vi "Treat Command.vi"(8 "error in (no error)":errorcluster, 11 "Channel in":refnum<class "ECHARPE_Channel.lvclass">) -> (0 "error out":errorcluster, 3 "Channel out":refnum<class "ECHARPE_Channel.lvclass">)   [LabVIEW 2018, in "ECHARPE_Channel.lvclass"]
doc: "Treat the commando received from the control interface."
uses:
  ECHARPE_Channel.lvclass
  C:/Users/Denis/Desktop/S4ACS/S4ACS/Channel/Channel.lvclass
  Channel/Channel.lvclass/Channel.ctl
  RxTx/RxTx.lvclass
  State Machine/State Machine.lvclass
  Sim_CCD/Sim_CCD.lvclass
  Channel/Channel.lvclass
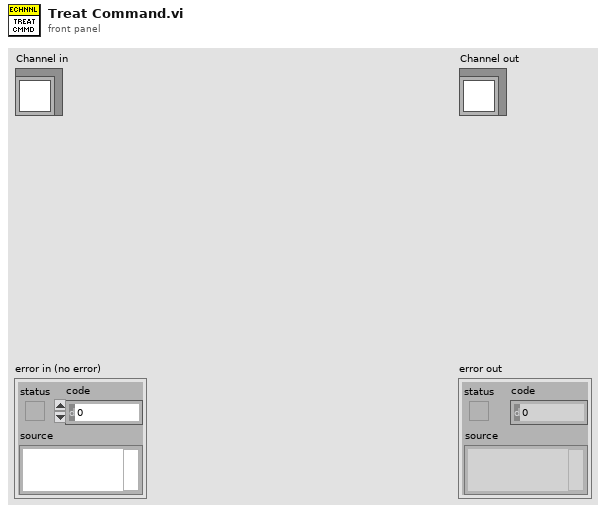
[diagram p1: front panel]
types:
  T1 = cluster{"State Machine.lvclass":refnum<class "State Machine.lvclass">, "RxTx.lvclass":refnum<class "RxTx.lvclass">, "Save_Header_RxTx.lvclass":refnum<class "RxTx.lvclass">, "Status SM.lvclass":refnum<class "State Machine.lvclass">, "Status RxTx.lvclass":refnum<class "RxTx.lvclass">, "servers array":refnum<class "Server.lvclass">[], "Events log file.lvclass":refnum<class "Log File.lvclass">, "Errors log file.lvclass":refnum<class "Log File.lvclass">, "Keywords log file.lvclass":refnum<class "Log File.lvclass">, "Sim_CCD.lvclass":refnum<class "Sim_CCD.lvclass">}
  T2 = cluster{"field 1":string, "field 2":string, "field 3":string}
  T3 = cluster{"Stop Acquisition":bool, "Abort Acquisition":bool, "Pause acquisition":bool, "wait expose command":bool, "video mode":bool, "stop app":bool}
  T4 = cluster{"FRAMES_DONE":u16, "CCD_STATUS":string, "CURRENT_TEMPERATURE":i16, "TEMPERATURE_STATUS":string, "FRAME_EXPOSURE_TIME":dbl, "SERIAL_NUMBER":u16, "ACQUIRING":bool, "POWER":bool, "ACS MODE":bool}
  T5 = cluster{"CYCLES_DONE":u16, "LAST_IMAGE_NAME":string, "USED_DISK_SPACE":u16, "IMAGE_INDEX":u32, "acquisition error":bool}
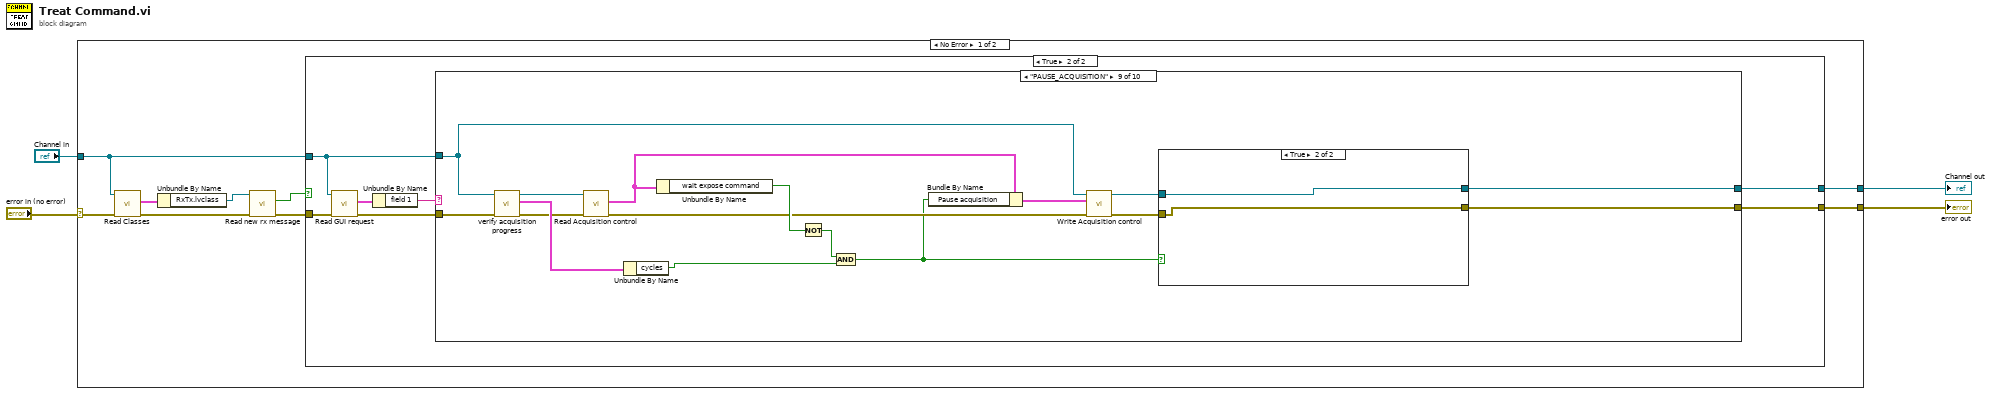
[diagram p0: block diagram]
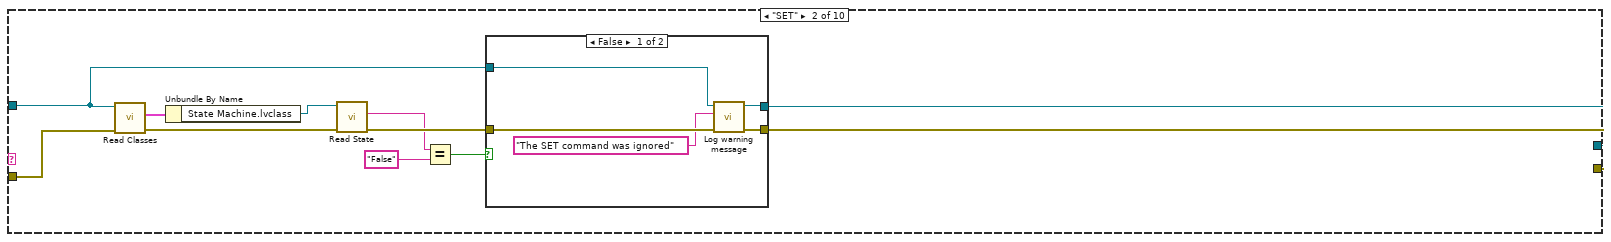
[diagram p4: hidden frame]
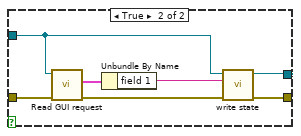
[diagram p5: hidden frame]
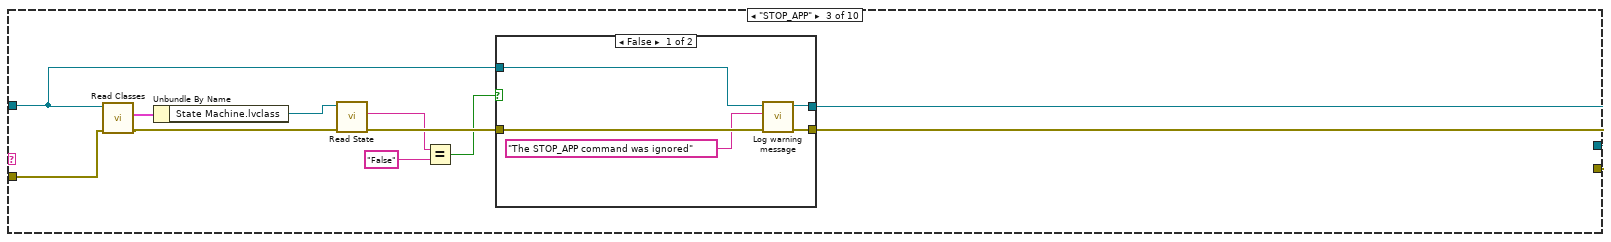
[diagram p6: hidden frame]
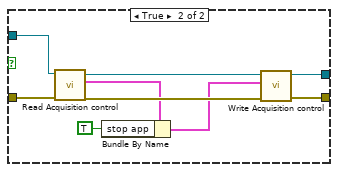
[diagram p7: hidden frame]
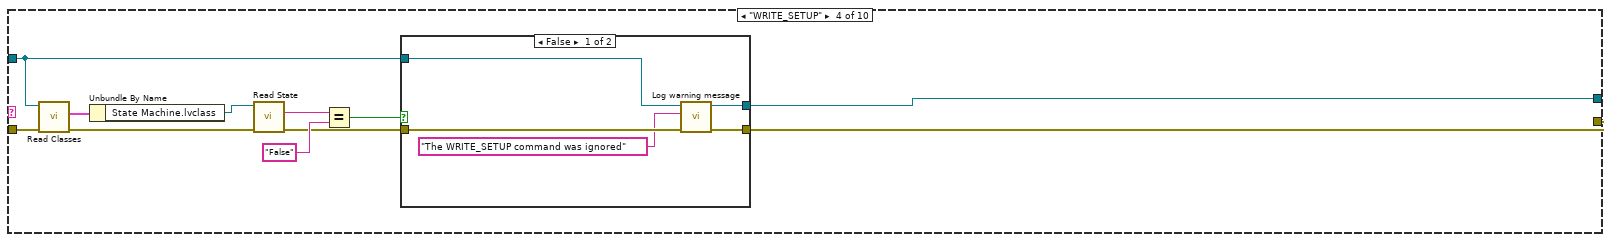
[diagram p8: hidden frame]
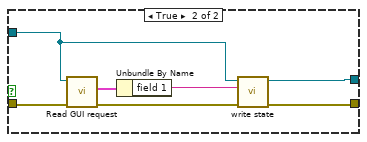
[diagram p9: hidden frame]
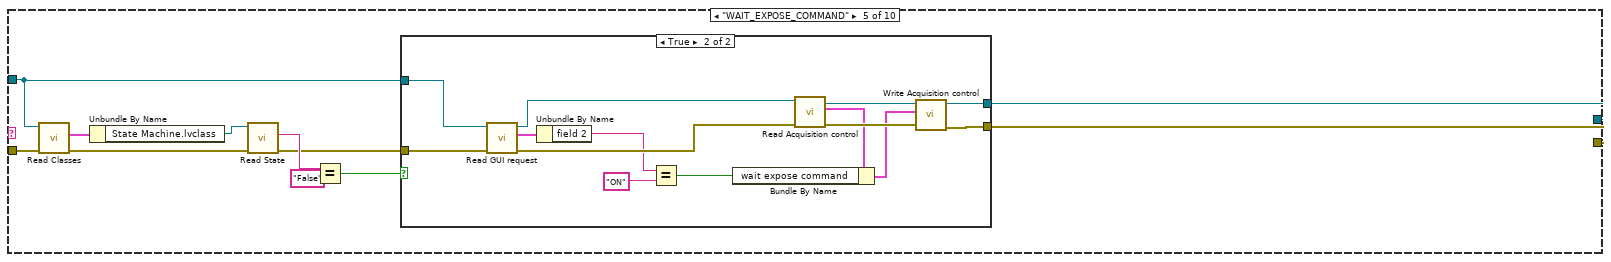
[diagram p10: hidden frame]
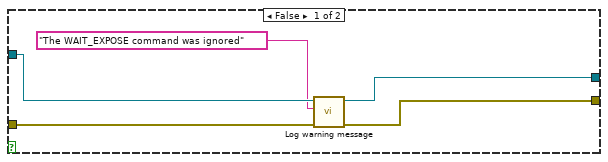
[diagram p11: hidden frame]
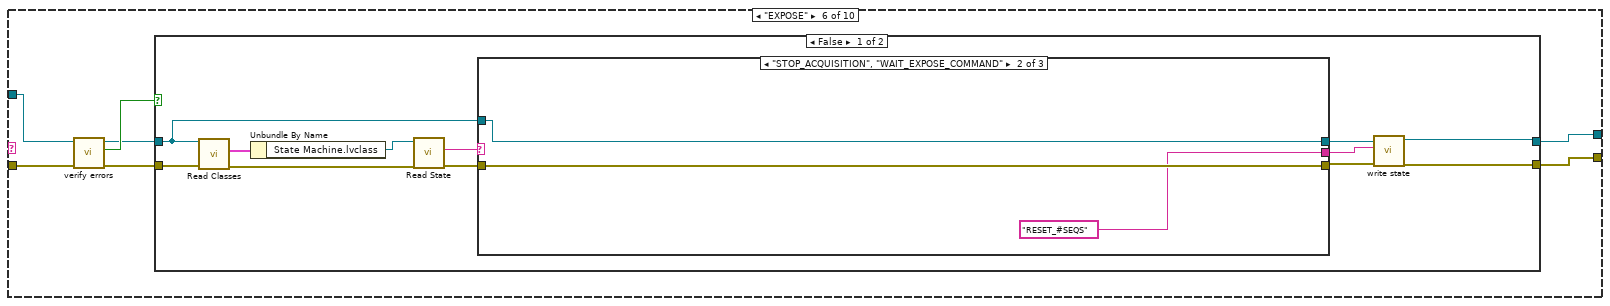
[diagram p12: hidden frame]
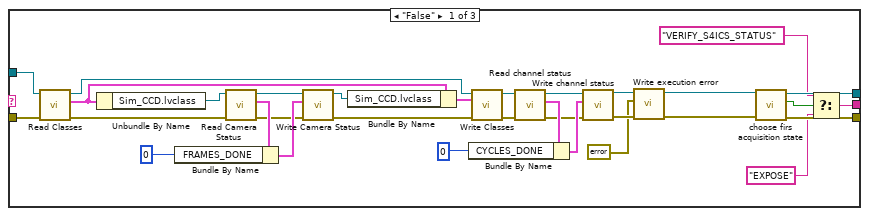
[diagram p13: hidden frame]
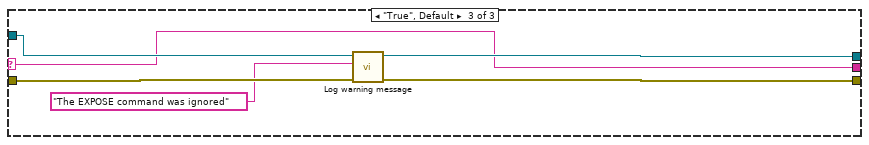
[diagram p14: hidden frame]
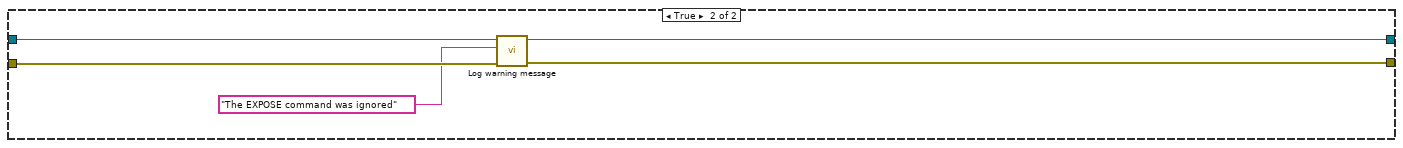
[diagram p15: hidden frame]
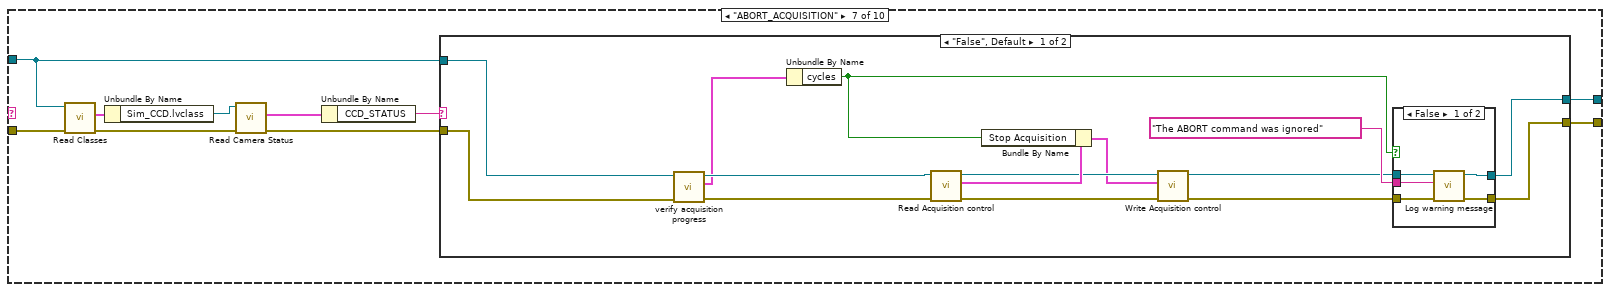
[diagram p16: hidden frame]
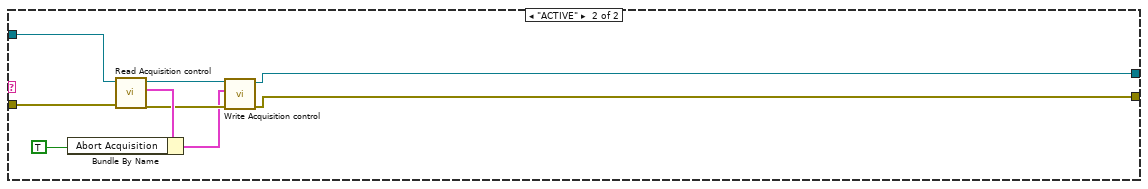
[diagram p18: hidden frame]
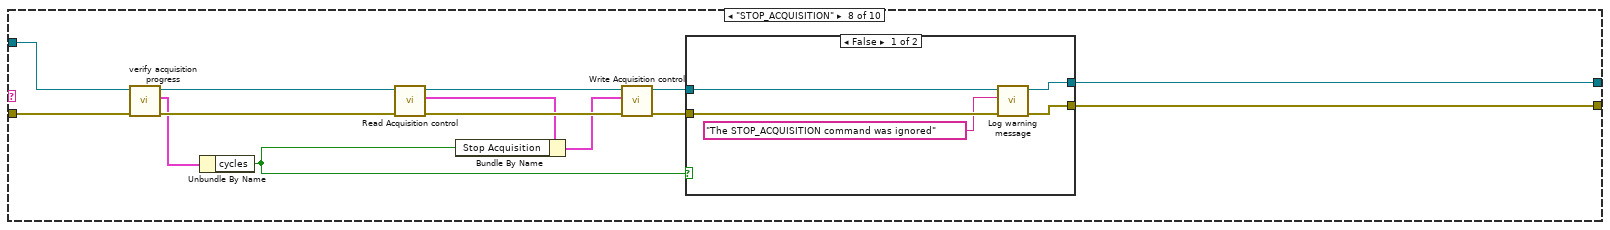
[diagram p19: hidden frame]
diagram:
  n1 = case shown="No Error" "error in (no error)" {
    selector: "error in (no error)" -> [w9 w299]
    tunnel: [w12 w299] -> w3
    tunnel: [w13 w298] -> w1
    tunnel: "Channel in" -> [w8 w298]
    frame No Error {
      n2 = call-dynamic "Read Classes.vi"("error in (no error)"=w9, "Channel in"=w8) -> ("error out"=w7:errorcluster, "Classes"=w6:T1)  [unwired: 7 in, 1 out]
      n3 = Unbundle By Name(w6) -> ("RxTx.lvclass"=w5:refnum<class "RxTx.lvclass">)
      n4 = call-dynamic "Read new rx message.vi"("error in (no error)"=w7, "RxTx in"=w5) -> ("error out"=w11:errorcluster, "new rx message"=w10:bool)  [unwired: 7 in, 1 out]
      n5 = case shown="True" w10 {
        tunnel: w11 -> [w14 w20]
        tunnel: [w15 w22] -> w13
        tunnel: [w14 w21] -> w12
        tunnel: w8 -> [w15 w19]
        frame False {
        }
        frame True {
          n6 = call "Read GUI request.vi"("error in (no error)"=w20, "Channel in"=w19) -> ("error out"=w18:errorcluster, "GUI request"=w17:T2)  [unwired: 7 in, 1 out]
          n7 = Unbundle By Name(w17) -> ("field 1"=w16:string)
          n8 = case shown="\"PAUSE_ACQUISITION\"" w16 {
            tunnel: w19 -> [w24 w29 w51 w76 w98 w129 w193 w240 w259 w284]
            tunnel: [w24 w33 w56 w80 w102 w131 w200 w245 w268 w290] -> w22
            tunnel: w18 -> [w23 w28 w50 w75 w99 w130 w194 w241 w260 w283]
            tunnel: [w23 w32 w55 w79 w101 w132 w196 w244 w267 w289] -> w21
            frame "False", Default {
            }
            frame "SET" {
              n9 = call-dynamic "Read Classes.vi"("error in (no error)"=w28, "Channel in"=w29) -> ("error out"=w27:errorcluster, "Classes"=w26:T1)  [unwired: 7 in, 1 out]
              n10 = Unbundle By Name(w26) -> ("State Machine.lvclass"=w25:refnum<class "State Machine.lvclass">)
              n11 = call-dynamic "Read State.vi"("error in (no error)"=w27, "State Machine in"=w25) -> ("error out"=w35:errorcluster, "State"=w31:string)  [unwired: 7 in, 1 out]
              n12 = Equal?(x=w31, y="False") -> (x = y?=w30:bool)
              n13 = case shown="False" w30 {
                tunnel: w35 -> [w40 w44]
                tunnel: [w38 w47] -> w33
                tunnel: [w39 w46] -> w32
                tunnel: w29 -> [w37 w42]
                frame False {
                  n14 = call "Log warning message.vi"("error in (no error)"=w40, "String"="The SET command was ignored", "Channel in"=w37) -> ("error out"=w39:errorcluster, "Channel out"=w38:refnum<class "ECHARPE_Channel.lvclass">)  [unwired: 7 in]
                }
                frame True {
                  n15 = call "Read GUI request.vi"("error in (no error)"=w44, "Channel in"=w42) -> ("error out"=w43:errorcluster, "GUI request"=w45:T2)  [unwired: 7 in, 1 out]
                  n16 = Unbundle By Name(w45) -> ("field 1"=w41:string)
                  n17 = call "write state.vi"("error in (no error)"=w43, "state"=w41, "Channel in"=w42) -> ("error out"=w46:errorcluster, "Channel out"=w47:refnum<class "ECHARPE_Channel.lvclass">)  [unwired: 7 in]
                }
              }
            }
            frame "STOP_APP" {
              n18 = call-dynamic "Read Classes.vi"("error in (no error)"=w50, "Channel in"=w51) -> ("error out"=w48:errorcluster, "Classes"=w52:T1)  [unwired: 7 in, 1 out]
              n19 = Unbundle By Name(w52) -> ("State Machine.lvclass"=w49:refnum<class "State Machine.lvclass">)
              n20 = call-dynamic "Read State.vi"("error in (no error)"=w48, "State Machine in"=w49) -> ("error out"=w58:errorcluster, "State"=w54:string)  [unwired: 7 in, 1 out]
              n21 = Equal?(x=w54, y="False") -> (x = y?=w53:bool)
              n22 = case shown="False" w53 {
                tunnel: w58 -> [w63 w70]
                tunnel: [w61 w72] -> w56
                tunnel: [w62 w71] -> w55
                tunnel: w51 -> [w60 w69]
                frame False {
                  n23 = call "Log warning message.vi"("error in (no error)"=w63, "String"="The STOP_APP command was ignored", "Channel in"=w60) -> ("error out"=w62:errorcluster, "Channel out"=w61:refnum<class "ECHARPE_Channel.lvclass">)  [unwired: 7 in]
                }
                frame True {
                  n24 = call "Read Acquisition control.vi"("error in (no error)"=w70, "Channel in"=w69) -> ("error out"=w67:errorcluster, "Acquisition control"=w66:T3, "Channel out"=w68:refnum<class "ECHARPE_Channel.lvclass">)  [unwired: 7 in]
                  n25 = Bundle By Name(cluster=w66, "stop app"=TRUE) -> (w65:T3)
                  n26 = call "Write Acquisition control.vi"("error in (no error)"=w67, "Acquisition control"=w65, "Channel in"=w68) -> ("error out"=w71:errorcluster, "Channel out"=w72:refnum<class "ECHARPE_Channel.lvclass">)  [unwired: 7 in]
                }
              }
            }
            frame "WRITE_SETUP" {
              n27 = call-dynamic "Read Classes.vi"("error in (no error)"=w75, "Channel in"=w76) -> ("error out"=w74:errorcluster, "Classes"=w77:T1)  [unwired: 7 in, 1 out]
              n28 = Unbundle By Name(w77) -> ("State Machine.lvclass"=w73:refnum<class "State Machine.lvclass">)
              n29 = call-dynamic "Read State.vi"("error in (no error)"=w74, "State Machine in"=w73) -> ("error out"=w81:errorcluster, "State"=w78:string)  [unwired: 7 in, 1 out]
              n30 = Equal?(x=w78, y="False") -> (x = y?=w82:bool)
              n31 = case shown="False" w82 {
                tunnel: w81 -> [w87 w92]
                tunnel: [w85 w90] -> w80
                tunnel: [w86 w89] -> w79
                tunnel: w76 -> [w88 w91]
                frame False {
                  n32 = call "Log warning message.vi"("error in (no error)"=w87, "String"="The WRITE_SETUP command was ignored", "Channel in"=w88) -> ("error out"=w86:errorcluster, "Channel out"=w85:refnum<class "ECHARPE_Channel.lvclass">)  [unwired: 7 in]
                }
                frame True {
                  n33 = call "Read GUI request.vi"("error in (no error)"=w92, "Channel in"=w91) -> ("error out"=w94:errorcluster, "GUI request"=w95:T2)  [unwired: 7 in, 1 out]
                  n34 = Unbundle By Name(w95) -> ("field 1"=w93:string)
                  n35 = call "write state.vi"("error in (no error)"=w94, "state"=w93, "Channel in"=w91) -> ("error out"=w89:errorcluster, "Channel out"=w90:refnum<class "ECHARPE_Channel.lvclass">)  [unwired: 7 in]
                }
              }
            }
            frame "WAIT_EXPOSE_COMMAND" {
              n36 = call-dynamic "Read Classes.vi"("error in (no error)"=w99, "Channel in"=w98) -> ("error out"=w96:errorcluster, "Classes"=w100:T1)  [unwired: 7 in, 1 out]
              n37 = Unbundle By Name(w100) -> ("State Machine.lvclass"=w97:refnum<class "State Machine.lvclass">)
              n38 = call-dynamic "Read State.vi"("error in (no error)"=w96, "State Machine in"=w97) -> ("error out"=w103:errorcluster, "State"=w105:string)  [unwired: 7 in, 1 out]
              n39 = Equal?(x=w105, y="False") -> (x = y?=w104:bool)
              n40 = case shown="True" w104 {
                tunnel: w98 -> [w111 w123]
                tunnel: w103 -> [w108 w122]
                tunnel: [w110 w121] -> w102
                tunnel: [w109 w120] -> w101
                frame False {
                  n41 = call "Log warning message.vi"("error in (no error)"=w108, "String"="The WAIT_EXPOSE command was ignored", "Channel in"=w111) -> ("error out"=w109:errorcluster, "Channel out"=w110:refnum<class "ECHARPE_Channel.lvclass">)  [unwired: 7 in]
                }
                frame True {
                  n42 = call "Read GUI request.vi"("error in (no error)"=w122, "Channel in"=w123) -> ("error out"=w119:errorcluster, "GUI request"=w124:T2, "Channel out"=w116:refnum<class "ECHARPE_Channel.lvclass">)  [unwired: 7 in]
                  n43 = Unbundle By Name(w124) -> ("field 2"=w112:string)
                  n44 = Equal?(x=w112, y="ON") -> (x = y?=w113:bool)
                  n45 = call "Read Acquisition control.vi"("error in (no error)"=w119, "Channel in"=w116) -> ("error out"=w118:errorcluster, "Acquisition control"=w115:T3, "Channel out"=w117:refnum<class "ECHARPE_Channel.lvclass">)  [unwired: 7 in]
                  n46 = Bundle By Name(cluster=w115, "wait expose command"=w113) -> (w114:T3)
                  n47 = call "Write Acquisition control.vi"("error in (no error)"=w118, "Acquisition control"=w114, "Channel in"=w117) -> ("error out"=w120:errorcluster, "Channel out"=w121:refnum<class "ECHARPE_Channel.lvclass">)  [unwired: 7 in]
                }
              }
            }
            frame "EXPOSE" {
              n48 = call-dynamic "verify errors.vi"("error in (no error)"=w130, "Channel in"=w129) -> ("error out"=w126:errorcluster, "error"=w128:bool, "Channel out"=w127:refnum<class "ECHARPE_Channel.lvclass">)  [unwired: 7 in]
              n49 = case shown="False" w128 {
                tunnel: [w140 w187] -> w132
                tunnel: w126 -> [w136 w189]
                tunnel: w127 -> [w133 w190]
                tunnel: [w141 w188] -> w131
                frame False {
                  n50 = call-dynamic "Read Classes.vi"("error in (no error)"=w136, "Channel in"=w133) -> ("error out"=w135:errorcluster, "Classes"=w137:T1)  [unwired: 7 in, 1 out]
                  n51 = Unbundle By Name(w137) -> ("State Machine.lvclass"=w134:refnum<class "State Machine.lvclass">)
                  n52 = call-dynamic "Read State.vi"("error in (no error)"=w135, "State Machine in"=w134) -> ("error out"=w143:errorcluster, "State"=w144:string)  [unwired: 7 in, 1 out]
                  n53 = case shown="\"STOP_ACQUISITION\", \"WAIT_EXPOSE_COMMAND\"" w144 {
                    selector: w144 -> [_ _ w180]
                    tunnel: w133 -> [w165 w178 w185]
                    tunnel: w143 -> [w166 w179 w182]
                    tunnel: [w172 w178 w184] -> w142
                    tunnel: [w171 w179 w183] -> w139
                    tunnel: [w168 "RESET_#SEQS" w180] -> w138
                    frame "False" {
                      n54 = call-dynamic "Read Classes.vi"("error in (no error)"=w166, "Channel in"=w165) -> ("error out"=w163:errorcluster, "Classes"=w158:T1, "Channel out"=w155:refnum<class "ECHARPE_Channel.lvclass">)  [unwired: 7 in]
                      n55 = Unbundle By Name(w158) -> ("Sim_CCD.lvclass"=w164:refnum<class "Sim_CCD.lvclass">)
                      n56 = call "Read Camera Status.vi"("error in (no error)"=w163, "CCDCamera in"=w164) -> ("error out"=w173:errorcluster, "camera status"=w175:T4, "CCDCamera out"=w176:refnum<class "Sim_CCD.lvclass">)  [unwired: 7 in]
                      n57 = Bundle By Name(cluster=w175, "FRAMES_DONE"=u16 0 ("CUBES_DONE")) -> (w174:T4)
                      n58 = call "Write Camera Status.vi"("error in (no error)"=w173, "camera status"=w174, "CCDCamera in"=w176) -> ("error out"=w159:errorcluster, "CCDCamera out"=w156:refnum<class "Sim_CCD.lvclass">)  [unwired: 7 in]
                      n59 = Bundle By Name(cluster=w158, "Sim_CCD.lvclass"=w156) -> (w157:T1)
                      n60 = call-dynamic "Write Classes.vi"("error in (no error)"=w159, "Classes"=w157, "Channel in"=w155) -> ("error out"=w154:errorcluster, "Channel out"=w153:refnum<class "ECHARPE_Channel.lvclass">)  [unwired: 7 in]
                      n61 = call-dynamic "Read channel status.vi"("error in (no error)"=w154, "Channel in"=w153) -> ("error out"=w151:errorcluster, "channel status"=w162:T5, "Channel out"=w152:refnum<class "ECHARPE_Channel.lvclass">)  [unwired: 7 in]
                      n62 = Bundle By Name(cluster=w162, "CYCLES_DONE"=u16 0 ("CUBES_DONE")) -> (w161:T5)
                      n63 = call-dynamic "Write channel status.vi"("error in (no error)"=w151, "channel status"=w161, "Channel in"=w152) -> ("error out"=w148:errorcluster, "Channel out"=w149:refnum<class "ECHARPE_Channel.lvclass">)  [unwired: 7 in]
                      n64 = call-dynamic "Write execution error.vi"("error in (no error)"=w148, "execution error"=errorcluster {"status"=FALSE, "code"=0, "source"=""}, "Channel in"=w149) -> ("error out"=w145:errorcluster, "Channel out"=w146:refnum<class "ECHARPE_Channel.lvclass">)  [unwired: 7 in]
                      n65 = call "choose firs acquisition state.vi"("error in (no error)"=w145, "Channel in"=w146) -> ("error out"=w171:errorcluster, "verify S4ICS status"=w167:bool, "Channel out"=w172:refnum<class "ECHARPE_Channel.lvclass">)  [unwired: 7 in]
                      n66 = Select(t="VERIFY_S4ICS_STATUS" ("x"), s=w167, f="EXPOSE" ("x")) -> (s? t:f=w168:string)
                    }
                    frame "STOP_ACQUISITION", "WAIT_EXPOSE_COMMAND" {
                    }
                    frame "True", Default {
                      n67 = call "Log warning message.vi"("error in (no error)"=w182, "String"="The EXPOSE command was ignored", "Channel in"=w185) -> ("error out"=w183:errorcluster, "Channel out"=w184:refnum<class "ECHARPE_Channel.lvclass">)  [unwired: 7 in]
                    }
                  }
                  n68 = call "write state.vi"("error in (no error)"=w139, "state"=w138, "Channel in"=w142) -> ("error out"=w140:errorcluster, "Channel out"=w141:refnum<class "ECHARPE_Channel.lvclass">)  [unwired: 7 in]
                }
                frame True {
                  n69 = call "Log warning message.vi"("error in (no error)"=w189, "String"="The EXPOSE command was ignored" ("Message to log"), "Channel in"=w190) -> ("error out"=w187:errorcluster, "Channel out"=w188:refnum<class "ECHARPE_Channel.lvclass">)  [unwired: 7 in]
                }
              }
            }
            frame "ABORT_ACQUISITION" {
              n70 = call-dynamic "Read Classes.vi"("error in (no error)"=w194, "Channel in"=w193) -> ("error out"=w191:errorcluster, "Classes"=w195:T1)  [unwired: 7 in, 1 out]
              n71 = Unbundle By Name(w195) -> ("Sim_CCD.lvclass"=w192:refnum<class "Sim_CCD.lvclass">)
              n72 = call "Read Camera Status.vi"("error in (no error)"=w191, "CCDCamera in"=w192) -> ("error out"=w197:errorcluster, "camera status"=w199:T4)  [unwired: 7 in, 1 out]
              n73 = Unbundle By Name(w199) -> ("CCD_STATUS"=w198:string)
              n74 = case shown="\"False\", Default" w198 {
                tunnel: w193 -> [w206 w225]
                tunnel: [w214 w224] -> w200
                tunnel: w197 -> [w205 w226]
                tunnel: [w213 w223] -> w196
                frame "False", Default {
                  n75 = call "verify acquisition progress.vi"("error in (no error)"=w205, "SPARC4_Channel in"=w206) -> ("error out"=w203:errorcluster, "acq in progress"=w202:cluster{"frames":bool, "cycles":bool}, "SPARC4_Channel out"=w204:refnum<class "ECHARPE_Channel.lvclass">)  [unwired: 7 in]
                  n76 = Unbundle By Name(w202) -> ("cycles"=w201:bool)
                  n77 = call "Read Acquisition control.vi"("error in (no error)"=w203, "Channel in"=w204) -> ("error out"=w210:errorcluster, "Acquisition control"=w212:T3, "Channel out"=w211:refnum<class "ECHARPE_Channel.lvclass">)  [unwired: 7 in]
                  n78 = Bundle By Name(cluster=w212, "Stop Acquisition"=w201) -> (w209:T3)
                  n79 = call "Write Acquisition control.vi"("error in (no error)"=w210, "Acquisition control"=w209, "Channel in"=w211) -> ("error out"=w207:errorcluster, "Channel out"=w208:refnum<class "ECHARPE_Channel.lvclass">)  [unwired: 7 in]
                  n80 = case shown="False" w201 {
                    tunnel: "The ABORT command was ignored" ("Message to log") -> [w220 _]
                    tunnel: w208 -> [w219 w221]
                    tunnel: [w218 w221] -> w214
                    tunnel: [w217 w222] -> w213
                    tunnel: w207 -> [w216 w222]
                    frame False {
                      n81 = call "Log warning message.vi"("error in (no error)"=w216, "String"=w220, "Channel in"=w219) -> ("error out"=w217:errorcluster, "Channel out"=w218:refnum<class "ECHARPE_Channel.lvclass">)  [unwired: 7 in]
                    }
                    frame True {
                    }
                  }
                }
                frame "ACTIVE" {
                  n82 = call "Read Acquisition control.vi"("error in (no error)"=w226, "Channel in"=w225) -> ("error out"=w229:errorcluster, "Acquisition control"=w231:T3, "Channel out"=w230:refnum<class "ECHARPE_Channel.lvclass">)  [unwired: 7 in]
                  n83 = Bundle By Name(cluster=w231, "Abort Acquisition"=TRUE) -> (w228:T3)
                  n84 = call "Write Acquisition control.vi"("error in (no error)"=w229, "Acquisition control"=w228, "Channel in"=w230) -> ("error out"=w223:errorcluster, "Channel out"=w224:refnum<class "ECHARPE_Channel.lvclass">)  [unwired: 7 in]
                }
              }
            }
            frame "STOP_ACQUISITION" {
              n85 = call "verify acquisition progress.vi"("error in (no error)"=w241, "SPARC4_Channel in"=w240) -> ("error out"=w237:errorcluster, "acq in progress"=w236:cluster{"frames":bool, "cycles":bool}, "SPARC4_Channel out"=w239:refnum<class "ECHARPE_Channel.lvclass">)  [unwired: 7 in]
              n86 = Unbundle By Name(w236) -> ("cycles"=w235:bool)
              n87 = call "Read Acquisition control.vi"("error in (no error)"=w237, "Channel in"=w239) -> ("error out"=w243:errorcluster, "Acquisition control"=w233:T3, "Channel out"=w238:refnum<class "ECHARPE_Channel.lvclass">)  [unwired: 7 in]
              n88 = Bundle By Name(cluster=w233, "Stop Acquisition"=w235) -> (w232:T3)
              n89 = call "Write Acquisition control.vi"("error in (no error)"=w243, "Acquisition control"=w232, "Channel in"=w238) -> ("error out"=w242:errorcluster, "Channel out"=w234:refnum<class "ECHARPE_Channel.lvclass">)  [unwired: 7 in]
              n90 = case shown="False" w235 {
                tunnel: w234 -> [w250 w252]
                tunnel: w242 -> [w249 w251]
                tunnel: [w247 w252] -> w245
                tunnel: [w248 w251] -> w244
                frame False {
                  n91 = call "Log warning message.vi"("error in (no error)"=w249, "String"="The STOP_ACQUISITION command was ignored", "Channel in"=w250) -> ("error out"=w248:errorcluster, "Channel out"=w247:refnum<class "ECHARPE_Channel.lvclass">)  [unwired: 7 in]
                }
                frame True {
                }
              }
            }
            frame "PAUSE_ACQUISITION" {
              n92 = call "verify acquisition progress.vi"("error in (no error)"=w260, "SPARC4_Channel in"=w259) -> ("error out"=w262:errorcluster, "acq in progress"=w265:cluster{"frames":bool, "cycles":bool}, "SPARC4_Channel out"=w261:refnum<class "ECHARPE_Channel.lvclass">)  [unwired: 7 in]
              n93 = call "Read Acquisition control.vi"("error in (no error)"=w262, "Channel in"=w261) -> ("error out"=w258:errorcluster, "Acquisition control"=w255:T3)  [unwired: 7 in, 1 out]
              n94 = Unbundle By Name(w265) -> ("cycles"=w264:bool)
              n95 = Unbundle By Name(w255) -> ("wait expose command"=w263:bool)
              n96 = Not(x=w263) -> (.not. x?=w266:bool)
              n97 = And(x=w266, y=w264) -> (x .and. y?=w254:bool)
              n98 = Bundle By Name(cluster=w255, "Pause acquisition"=w254) -> (w253:T3)
              n99 = call "Write Acquisition control.vi"("error in (no error)"=w258, "Acquisition control"=w253, "Channel in"=w259) -> ("error out"=w257:errorcluster, "Channel out"=w256:refnum<class "ECHARPE_Channel.lvclass">)  [unwired: 7 in]
              n100 = case shown="True" w254 {
                tunnel: w256 -> [w273 w275]
                tunnel: w257 -> [w272 w274]
                tunnel: [w270 w275] -> w268
                tunnel: [w271 w274] -> w267
                frame False {
                  n101 = call "Log warning message.vi"("error in (no error)"=w272, "String"="The PAUSE_ACQUISITION command was ignored", "Channel in"=w273) -> ("error out"=w271:errorcluster, "Channel out"=w270:refnum<class "ECHARPE_Channel.lvclass">)  [unwired: 7 in]
                }
                frame True {
                }
              }
            }
            frame "RESUME_ACQUISITION" {
              n102 = call "Read Acquisition control.vi"("error in (no error)"=w283, "Channel in"=w284) -> ("error out"=w282:errorcluster, "Acquisition control"=w277:T3, "Channel out"=w281:refnum<class "ECHARPE_Channel.lvclass">)  [unwired: 7 in]
              n103 = Unbundle By Name(w277) -> ("Pause acquisition"=w287:bool, "wait expose command"=w288:bool)
              n104 = Bundle By Name(cluster=w277, "Pause acquisition"=FALSE ("Acquisition control.Pause acquisition")) -> (w278:T3)
              n105 = Not(x=w287) -> (.not. x?=w286:bool)
              n106 = call "Write Acquisition control.vi"("error in (no error)"=w282, "Acquisition control"=w278, "Channel in"=w281) -> ("error out"=w279:errorcluster, "Channel out"=w280:refnum<class "ECHARPE_Channel.lvclass">)  [unwired: 7 in]
              n107 = Or(x=w286, y=w288) -> (x .or. y?=w285:bool)
              n108 = case shown="True" w285 {
                tunnel: w280 -> [w292 w297]
                tunnel: w279 -> [w291 w296]
                tunnel: [w292 w294] -> w290
                tunnel: [w291 w295] -> w289
                frame False {
                }
                frame True {
                  n109 = call "Log warning message.vi"("error in (no error)"=w296, "String"="The RESUME_ACQUISITION command was ignored", "Channel in"=w297) -> ("error out"=w295:errorcluster, "Channel out"=w294:refnum<class "ECHARPE_Channel.lvclass">)  [unwired: 7 in]
                }
              }
            }
          }
        }
      }
    }
    frame Error {
    }
  }
  "error out" <- w3
  "Channel out" <- w1
